vi "Create All Message Queues.vi"(8 "error in (no error)":errorcluster) -> (0 "error out":errorcluster, 3 "Message Queues out":T1)   [LabVIEW 2015, in "Message Queue.lvlib"]
doc: "This VI creates and initializes all the message queues for your application. If your application requires more than one message queue, right-click the \"Message Queues\" constant above and select Open Type Def. Add the new Message Queue(s) to the type definition, then initialize them in this VI."
uses:
  Message Queue.lvlib
  All Message Queues.ctl
  Message Cluster.ctl
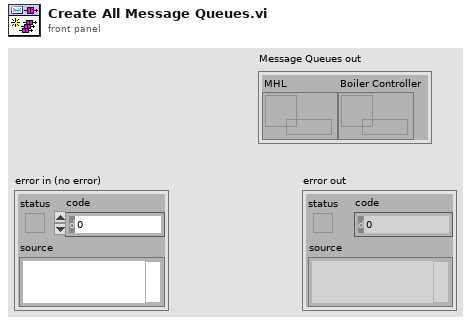
[diagram p1: front panel]
types:
  T1 = typedef "Message Queue.lvlib/All Message Queues.ctl" = cluster{"MHL":refnum<queue>, "Boiler Controller":refnum<queue>}
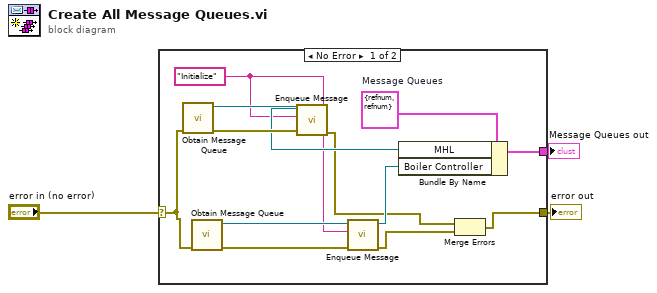
[diagram p0: block diagram]
diagram:
  n1 = case shown="No Error" "error in (no error)" {
    selector: "error in (no error)" -> [w12 w17]
    tunnel: [w15 _] -> w3
    tunnel: [w4 w17] -> w1
    frame No Error {
      w7 = "Initialize" ("Message")
      w16 = T1 {"MHL"=refnum, "Boiler Controller"=refnum}  # Message Queues
      n2 = call "Obtain Message Queue.vi"("error in (no error)"=w12) -> ("error out"=w11:errorcluster, "Message Queue"=w8:refnum<queue>)  [unwired: 9 in]
      n3 = call "Obtain Message Queue.vi"("error in (no error)"=w12) -> ("error out"=w14:errorcluster, "Message Queue"=w13:refnum<queue>)  [unwired: 9 in]
      n4 = call "Enqueue Message.vi"("error in (no error)"=w11, "Message"=w7, "Message Queue"=w8) -> ("error out"=w5:errorcluster, "dup Message Queue"=w9:refnum<queue>)  [unwired: 7 in]
      n5 = call "Enqueue Message.vi"("error in (no error)"=w14, "Message"=w7, "Message Queue"=w13) -> ("error out"=w6:errorcluster, "dup Message Queue"=w10:refnum<queue>)  [unwired: 7 in]
      n6 = Bundle By Name(cluster=w16, "MHL"=w9, "Boiler Controller"=w10) -> (w15:T1)
      n7 = Merge Errors(w5, w6) -> (w4:errorcluster)
    }
    frame Error {
    }
  }
  "Message Queues out" <- w3
  "error out" <- w1
